vi "Resolve Client Wrapper gRPC Dependencies.vi"(6 "Proto Names":T1, 8 "error in":errorcluster, 9 "New Subname":string, 10 "Template Project Path":path, 11 "Map - LibRef":map{string, refnum<vi>}(c390)) -> (0 "error out":errorcluster)   [LabVIEW 2021, in "Plugin Generator.lvlib"]
uses:
  Plugin Generator.lvlib
  Typedef/Proto Names.ctl
  <vilib>/CIF Foundation/CIF LabVIEW Scripting/LV Scripting/Typedef/Errors.ctl
  <vilib>/CIF Foundation/CIF Utilities/Errors/Append Error Location.vi
  <vilib>/CIF Foundation/CIF LabVIEW Scripting/LV Scripting/LV Scripting Utilities.lvlib
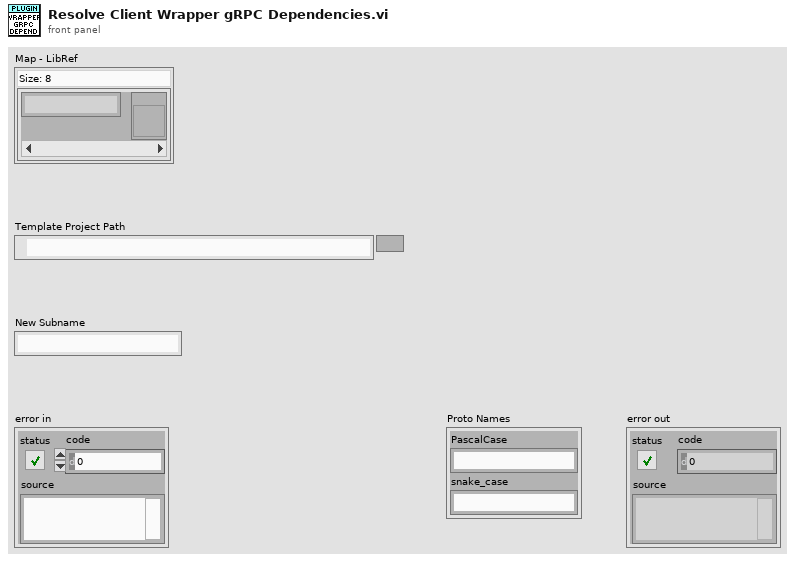
[diagram p1: front panel]
types:
  T1 = typedef "Plugin Generator.lvlib/Proto Names.ctl" = cluster{"PascalCase":string, "snake_case":string}
  T2 = typedef "Errors.ctl" = enum16{"Missing Version Changes", "Item not found"}
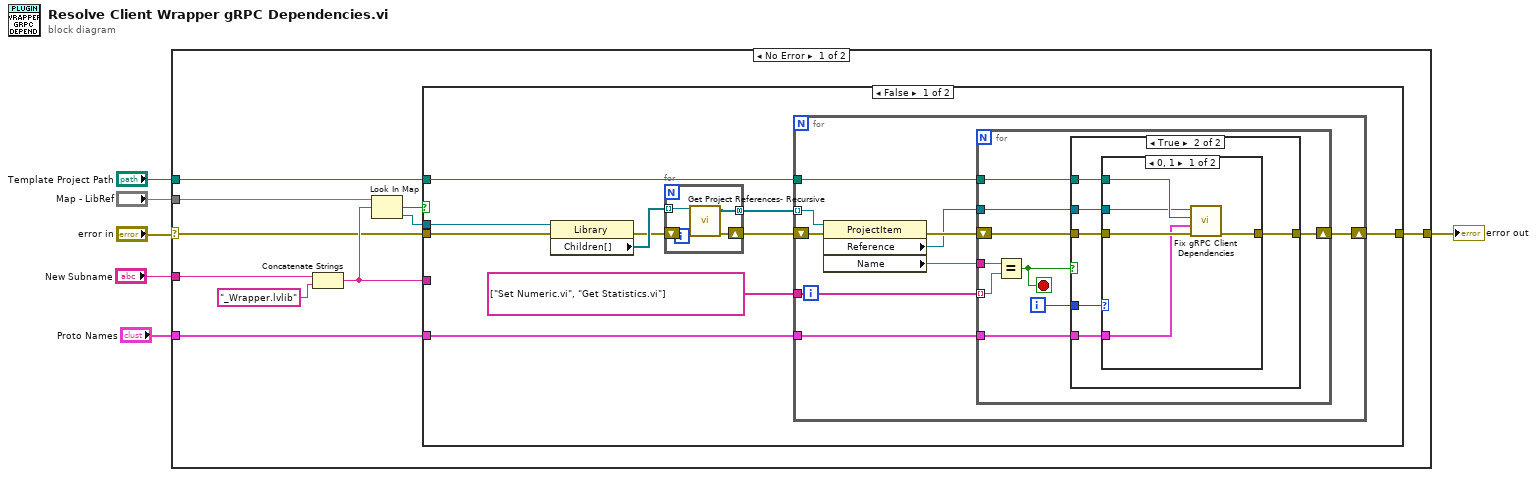
[diagram p0: block diagram]
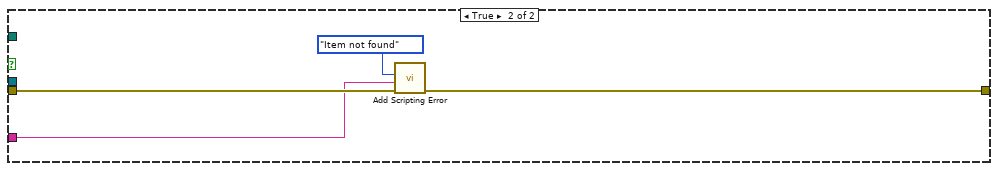
[diagram p4: hidden frame]
diagram:
  n1 = case shown="No Error" "error in" {
    selector: "error in" -> [w9 w66]
    tunnel: [w16 w66] -> w6
    tunnel: "Map - LibRef" -> [w12 _]
    tunnel: "Proto Names" -> [w7 _]
    tunnel: "Template Project Path" -> [w10 _]
    tunnel: "New Subname" -> [w8 _]
    frame No Error {
      n2 = Concatenate Strings(w8, "_Wrapper.lvlib" ("String")) -> (w11:string)
      n3 = Look In Map(map=w12, key=w11) -> (key not found?=w14:bool, value=w15:refnum<vi>)  [unwired: 1 in]
      n4 = case shown="False" w14 {
        tunnel: w15 -> [w26 _]
        tunnel: [w20 w63] -> w16
        tunnel: w7 -> [w21 _]
        tunnel: w11 -> [_ w62]
        tunnel: w10 -> [w19 _]
        tunnel: w9 -> [w17 w64]
        frame False {
          n5 = property class="Library"(reference=w26, error in=w17) -> (error out=w24:errorcluster, "Children[]"=w25:refnum<vi>[])  [unwired: 1 out]
          n6 = for {
            tunnel: w25 -> [w61] mode=indexing
            tunnel: [w60] -> w23 mode=concatenating
            shift-right: [w58] -> w18
            shift-left: w24 -> [w59]
            n7 = call <vilib>:"Get Project References- Recursive.vi"("error in"=w59, "TargetItem in"=w61) -> ("error out"=w58:errorcluster, "TargetItem out"=w60:refnum<vi>[])  [unwired: 8 in]
          }
          n8 = for {
            tunnel: w23 -> [w35] mode=indexing
            tunnel: string[] ["Set Numeric.vi", "Get Statistics.vi"] -> [w34]
            tunnel: w19 -> [w30]
            tunnel: w21 -> [w29]
            shift-right: [w28] -> w20
            shift-left: w18 -> [w33]
            n9 = property class="ProjectItem"(reference=w35, error in=w33) -> (error out=w32:errorcluster, "Reference"=w31:refnum<vi>, "Name"=w27:string)  [unwired: 1 out]
            n10 = for {
              tunnel: w34 -> [w44] mode=indexing
              tunnel: w27 -> [w43]
              tunnel: w31 -> [w41]
              tunnel: w30 -> [w38]
              tunnel: w29 -> [w37]
              shift-right: [w36] -> w28
              shift-left: w32 -> [w42]
              i -> [w39]
              stop <- w40 stop-if-true
              n11 = Equal?(x=w43, y=w44) -> (x = y?=w40:bool)
              n12 = case shown="True" w40 {
                tunnel: w42 -> [w45 w50]
                tunnel: w41 -> [_ w51]
                tunnel: w39 -> [_ w49]
                tunnel: w38 -> [_ w48]
                tunnel: w37 -> [_ w47]
                tunnel: [w45 w46] -> w36
                frame False {
                }
                frame True {
                  n13 = case shown="0, 1" w49 {
                    tunnel: w51 -> [w52 _]
                    tunnel: w50 -> [w56 w57]
                    tunnel: w48 -> [w53 _]
                    tunnel: w47 -> [w54 _]
                    tunnel: [w55 w57] -> w46
                    frame 0, 1 {
                      n14 = call "Fix gRPC Client Dependencies.vi"("error in"=w56, "Proto Names"=w54, "Project Path"=w53, "VI Refnum"=w52) -> ("error out"=w55:errorcluster)  [unwired: 7 in]
                    }
                    frame 3, Default {
                    }
                  }
                }
              }
            }
          }
        }
        frame True {
          n15 = call <vilib>:"Add Scripting Error.vi"("error in (no error)"=w64, "String to Append"=w62, "Error"=Errors."Item not found") -> ("error out"=w63:errorcluster)  [unwired: 8 in]
        }
      }
    }
    frame Error {
    }
  }
  "error out" <- w6
